vi "FW_image_naming.vi"(10 "Numeric":i32, 11 "Enum":T1) -> (3 "String":string)   [LabVIEW 2021, in "Framework_lib.lvlib"]
uses:
  QMH/Framework_lib.lvlib
  QMH/QMH_references_enum.ctl
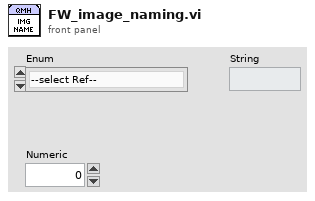
[diagram p1: front panel]
types:
  T1 = typedef "Framework_lib.lvlib/QMH_references_enum.ctl" = enum16{"--select Ref--", "Consumer_SUT", "Consumer_Annot", "Compute_Results"}
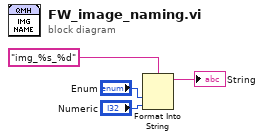
[diagram p0: block diagram]
diagram:
  n1 = Format Into String(format string="img_%s_%d", "Enum", "Numeric") -> (resulting string=→"String":string)  [unwired: 2 in, 1 out]
